vi "Close.vi"(8 "error in":errorcluster, 11 "Voltage Limit in":refnum<class "Voltage Limit.lvclass">) -> (0 "error out":errorcluster, 3 "Voltage Limit out":refnum<class "Voltage Limit.lvclass">)   [LabVIEW 2023, in "Voltage Limit.lvclass"]
uses:
  Voltage Limit.lvclass
  Parents/Limit/Limit.lvclass
  Voltage Limit.lvclass/Voltage Limit.ctl
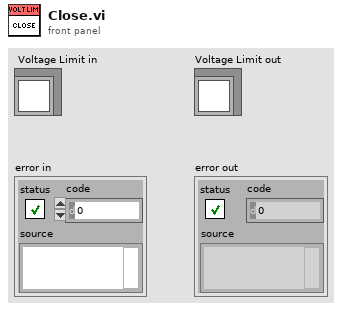
[diagram p1: front panel]
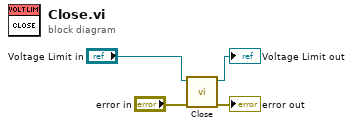
[diagram p0: block diagram]
diagram:
  n1 = call-parent "Close.vi"("error in"="error in", "Limit in"="Voltage Limit in") -> ("error out"=→"error out":errorcluster, "Limit out"=→"Voltage Limit out":refnum<class "Voltage Limit.lvclass">)  [unwired: 8 in]
